vi "Calc Torque.vi"(11 "MCU_I_s_q":dbl) -> (3 "Torque":dbl format="%#_g Nm")   [LabVIEW 2023, in "HSU MCU V2 CFG.lvclass"]
uses:
  HSU MCU V2 CFG.lvclass
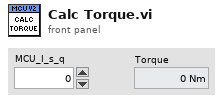
[diagram p1: front panel]
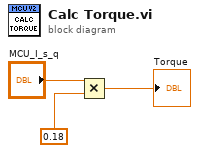
[diagram p0: block diagram]
diagram:
  n1 = Multiply(x="MCU_I_s_q", y=0.18) -> (x*y=→"Torque":dbl)
